vi "FRCts20_WebMethods_ReadData_Teams.vi"(8 "error in (no error)":errorcluster, 10 "Team In":T1, 11 "httpRequestID":u32) -> (0 "error out":errorcluster, 2 "Team In":T1, 3 "httpRequestID out":u32)   [LabVIEW 2014, in "FRCts20_WebMethods.lvlib"]
uses:
  FRCts20_WebMethods.lvlib
  <vilib>/wsapi/NI_WebServices.lvlib
  Backend/source/VI Source/FRCts20_Backend_API/FRCts20_Backend_API_Status.ctl
  Backend/source/VI Source/FRCts20_Backend_API/FRCts20_Backend_API_SW.ctl
  Backend/source/VI Source/FRCts20_Backend_API/FRCts20_Backend_API_Team.ctl
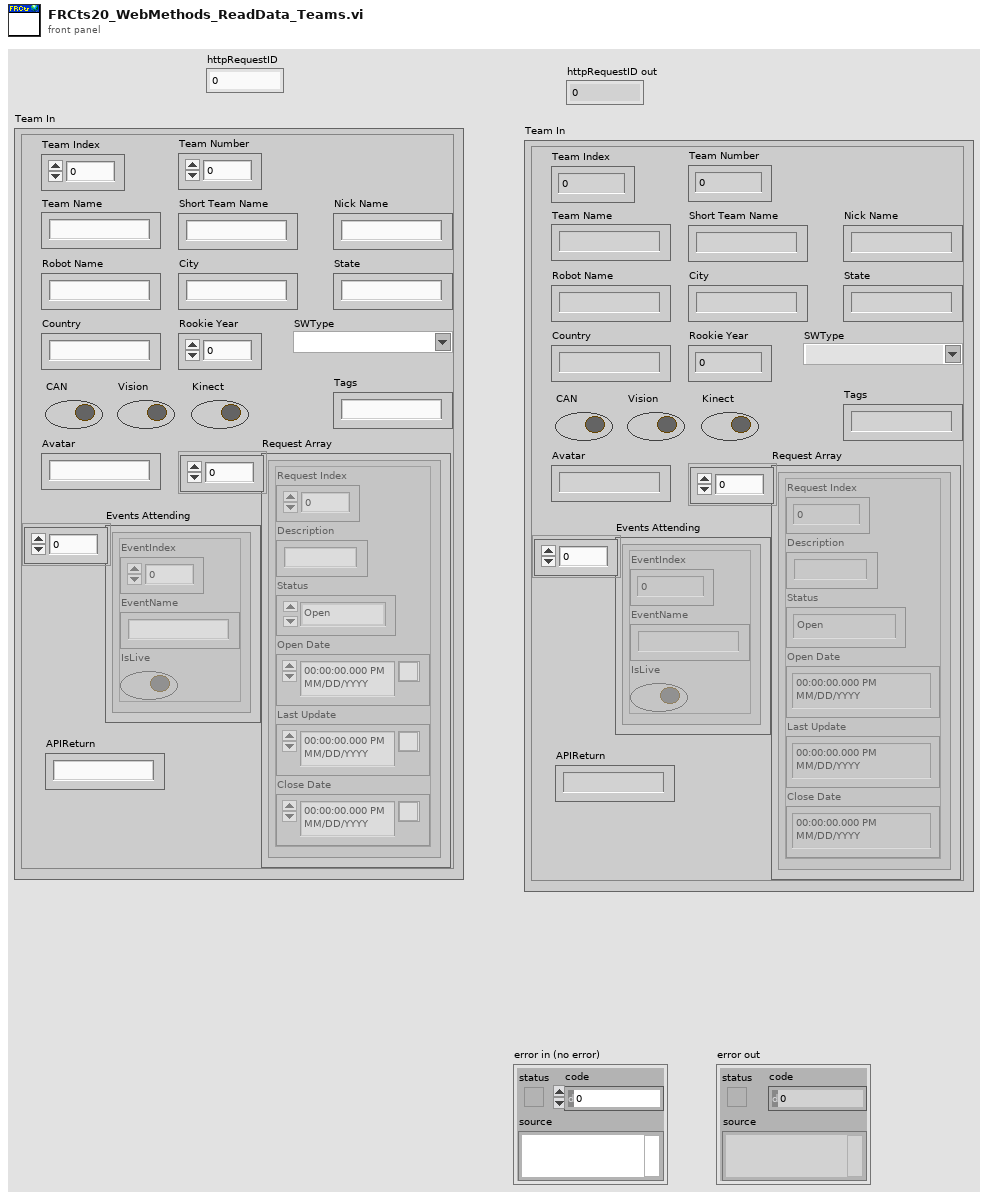
[diagram p1: front panel]
types:
  T1 = typedef "FRCts20_Backend_API.lvlib/FRCts20_Backend_API_Team.ctl" = cluster{"Team Index":u32, "Team Number":u32, "Team Name":string, "Short Team Name":string, "Nick Name":string, "Robot Name":string, "City":string, "State":string, "Country":string, "Rookie Year":u32, "SWType":T2, "CAN":bool, "Vision":bool, "Kinect":bool, "Tags":string, "Avatar":string, "Request Array":cluster{"Request Index":u32, "Description":string, "Status":T3, "Open Date":timestamp, "Last Update":timestamp, "Close Date":timestamp}[], "Events Attending":cluster{"EventIndex":dbl, "EventName":string, "IsLive":bool}[], "APIReturn":string}
  T2 = typedef "FRCts20_Backend_API.lvlib/FRCts20_Backend_API_SW.ctl" = string
  T3 = typedef "FRCts20_Backend_API.lvlib/FRCts20_Backend_API_Status.ctl" = enum16{"Open", "In Work", "Closed"}
  T4 = typedef "FRCts20_WebMethods.lvlib/FRCts20_WebMethods_ctl_returntype.ctl" = string
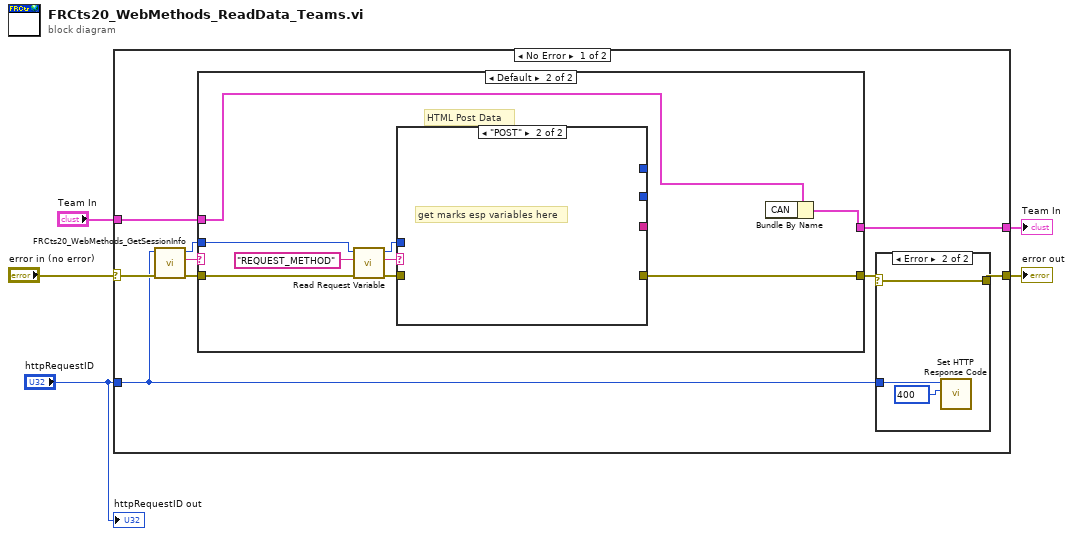
[diagram p0: block diagram]
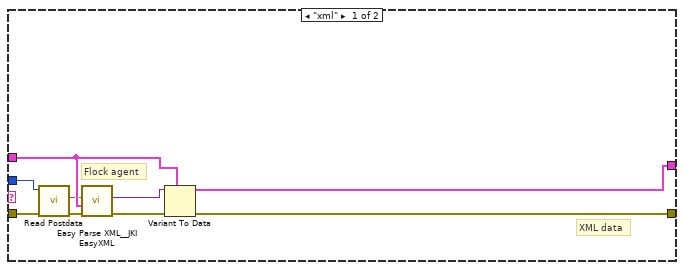
[diagram p3: hidden frame]
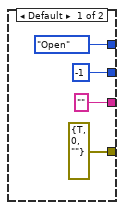
[diagram p4: hidden frame]
diagram:
  n1 = case shown="No Error" "error in (no error)" {
    selector: "error in (no error)" -> [w9 w42]
    tunnel: "httpRequestID" -> [w8 _]
    tunnel: "Team In" -> [w14 w41]
    tunnel: [w11 w42] -> w4
    tunnel: [w12 w41] -> w1
    frame No Error {
      n2 = call "FRCts20_WebMethods_GetSessionInfo.vi"("error in"=w9, "httpRequestID"=w8) -> ("error out"=w10:errorcluster, "Return Type"=w7:T4, "httpRequestID out"=w6:u32)  [unwired: 7 in]
      n3 = case shown="Default" w7 {
        tunnel: w10 -> [w22 w32]
        tunnel: w14 -> [w25 w35]
        tunnel: [w24 w36] -> w13
        tunnel: [w23 w34] -> w12
        tunnel: w6 -> [w19 w28]
        frame "xml" {
          # "Flock agent"
          # "XML data"
          n4 = call <vilib>:"Read Postdata.vi"("error in (no error)"=w22, "httpRequestID"=w19) -> ("error out"=w21:errorcluster, "postdata"=w20:string)  [unwired: 7 in, 1 out]
          n5 = call <vilib>:"Easy Parse XML__JKI EasyXML.vi"("error in (no error)"=w21, "LabVIEW Data (Type)"=w25, "XML String"=w20) -> ("error out"=w27:errorcluster, "LabVIEW Data"=w26:variant)  [unwired: 7 in]
          n6 = Variant To Data(error in=w27, type=w25, Variant=w26) -> (data=w23:T1, error out=w24:errorcluster)
        }
        frame Default {
          # "HTML Post Data"
          n7 = call <vilib>:"Read Request Variable.vi"("error in (no error)"=w32, "variable name"="REQUEST_METHOD", "httpRequestID"=w28) -> ("error out"=w31:errorcluster, "value"=w30:string, "httpRequestID out"=w29:u32)  [unwired: 6 in]
          n8 = case shown="\"POST\"" w30 {
            tunnel: [errorcluster {"status"=TRUE, "code"=0, "source"=""} ("error out") _] -> w36
            tunnel: ["" ("value") _] -> _
            tunnel: [-1 _] -> _
            tunnel: [FRCts20_Backend_API_Status."Open" ("Status") _] -> _
            tunnel: w31 -> [_ _]
            tunnel: w29 -> [_ _]
            frame Default {
            }
            frame "POST" {
              # "get marks esp variables here"
            }
          }
          n9 = Bundle By Name(cluster=w35) -> (w34:T1)  [unwired: 1 in]
        }
      }
      n10 = case shown="Error" w13 {
        selector: w13 -> [w15 w16]
        tunnel: [w15 w16] -> w11
        tunnel: w8 -> [_ w17]
        frame No Error {
        }
        frame Error {
          w18 = 400 items=["100"=100, "101"=101, "200"=200, "201"=201, "202"=202, "203"=203, "204"=204, "205"=205, "206"=206, "300"=300, "301"=301, "302"=302, "303"=303, "304"=304, "305"=305, "306"=306, "307"=307, "400"=400, "401"=401, "402"=402, "403"=403, "404"=404, "405"=405, "406"=406, "407"=407, "408"=408, "409"=409, "410"=410, "411"=411, "412"=412, "413"=413, "414"=414, "415"=415, "416"=416, "417"=417, "500"=500, "501"=501, "502"=502, "503"=503, "504"=504, "505"=505] ("response code (200)")
          n11 = call <vilib>:"Set HTTP Response Code.vi"("response code (200)"=w18, "httpRequestID"=w17) -> ()  [unwired: 8 in, 2 out]
        }
      }
    }
    frame Error {
    }
  }
  "Team In" <- w1
  "error out" <- w4
  "httpRequestID out" <- "httpRequestID"
